vi "MSEncoder Case-12-ResetRFCycle.vi"(8 "error in (no error)":errorcluster, 9 "ParamValIn":variant, 11 "MSEncoder in":refnum<class "MSEncoder.lvclass">) -> (0 "error out":errorcluster, 3 "MSEncoder out":refnum<class "MSEncoder.lvclass">)   [LabVIEW 2018, in "MSEncoder.lvclass"]
uses:
  MSEncoder.lvclass
  Ctl/MSEditorParam resetRFCycle.ctl
  MSEncoder.lvclass/MSEncoder.ctl
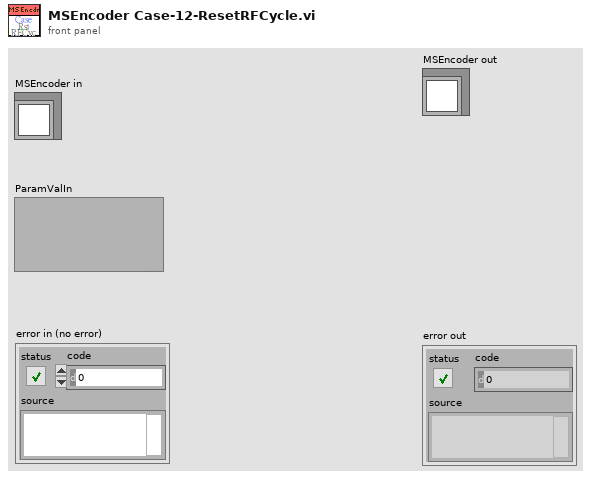
[diagram p1: front panel]
types:
  T1 = typedef "MSEditorParam resetRFCycle.ctl" = cluster{"iniPhase":u32}
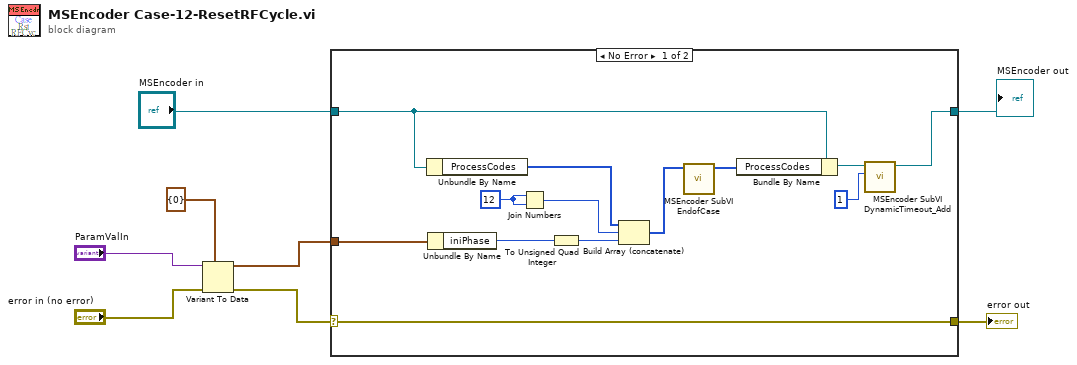
[diagram p0: block diagram]
diagram:
  n1 = Variant To Data(error in="error in (no error)", type=T1 {"iniPhase"=0} ("ParamValueType"), Variant="ParamValIn") -> (data=w3:T1, error out=w2:errorcluster)
  n2 = case shown="No Error" w2 {
    selector: w2 -> [w15 w23]
    tunnel: "MSEncoder in" -> [w20 w22]
    tunnel: [w15 w23] -> w8
    tunnel: [w12 w22] -> w7
    tunnel: w3 -> [w14 _]
    frame No Error {
      w18 = u32 12
      n3 = Unbundle By Name(w20) -> ("ProcessCodes"=w21:u64[])
      n4 = Unbundle By Name(w14) -> ("iniPhase"=w10:u32)
      n5 = Join Numbers(hi=w18, lo=w18) -> ((hi.lo)=w17:u64)
      n6 = To Unsigned Quad Integer(1:w10) -> (0:w9:u64)
      n7 = Build Array (concatenate)(w21, w17, w9) -> (w16:u64[])
      n8 = call "MSEncoder SubVI EndofCase.vi"("Case codes"=w16) -> ("Case codes with end"=w19:u64[])  [unwired: 9 in, 1 out]
      n9 = Bundle By Name(cluster=w20, "ProcessCodes"=w19) -> (w13:refnum<class "MSEncoder.lvclass">)
      n10 = call "MSEncoder SubVI DynamicTimeout_Add.vi"("Timeout_ms"=1, "MSEncoder"=w13) -> ("MSEncoder"=w12:refnum<class "MSEncoder.lvclass">)  [unwired: 8 in, 1 out]
    }
    frame Error {
    }
  }
  "error out" <- w8
  "MSEncoder out" <- w7
